vi "PAN_ModCaller.vi"(0 "CmdStringIn":string, 1 "modpath":path, 11 "error in (no error)":errorcluster) -> (4 "ImmedReplyString":string, 6 "new mod":bool, 15 "error out":errorcluster)   [LabVIEW 2016]
panel:
  in  "AVAPP Cmd Proc":refnum<vi>
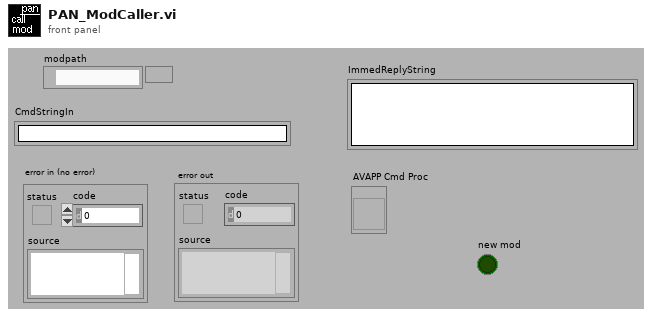
[diagram p1: front panel]
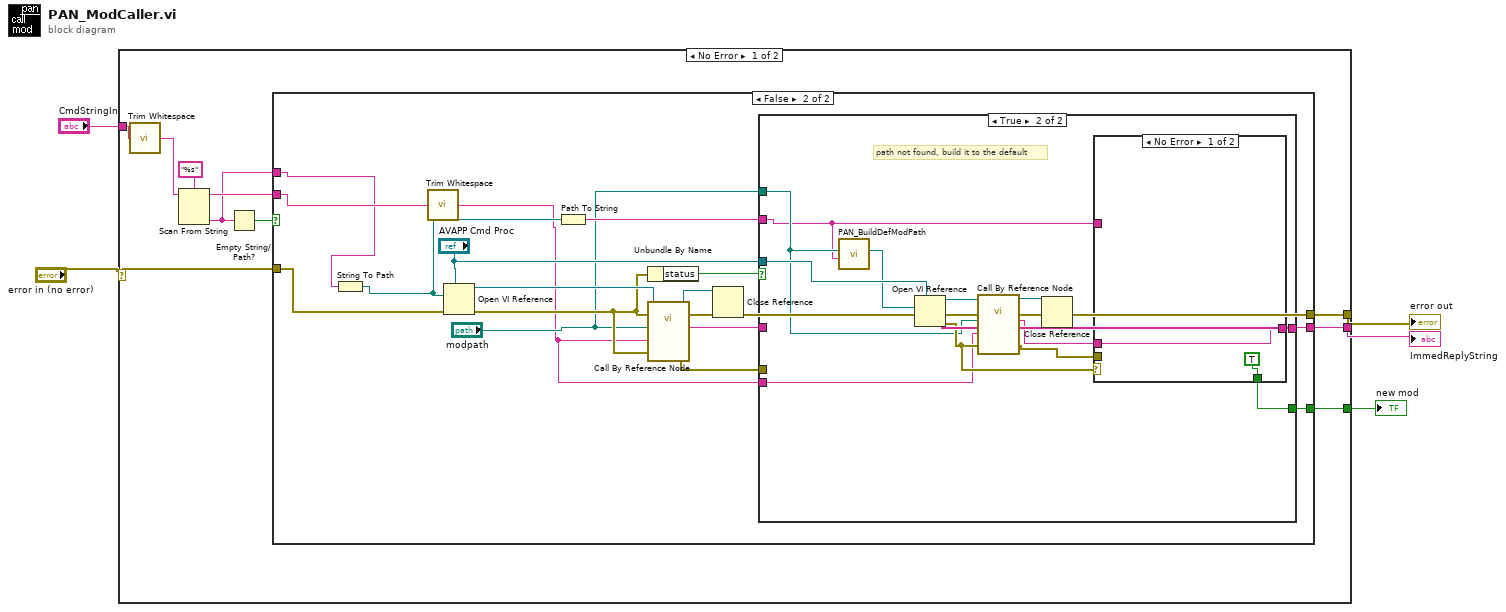
[diagram p0: block diagram]
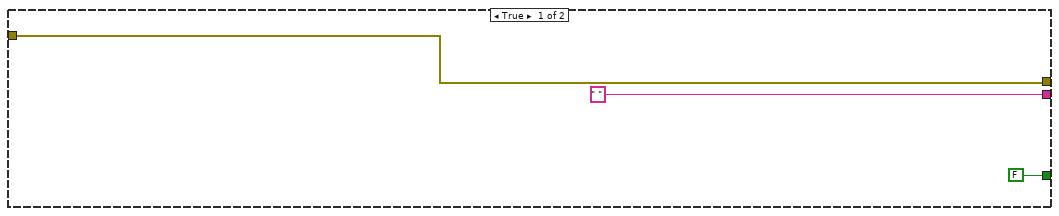
[diagram p2: hidden frame]
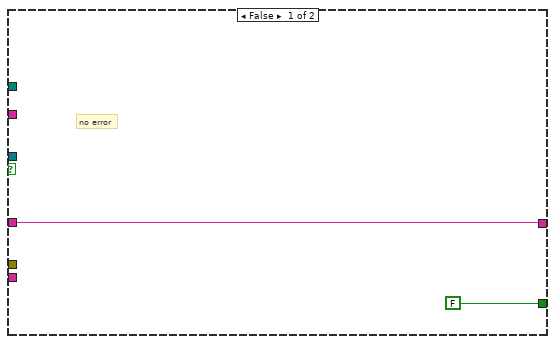
[diagram p3: hidden frame]
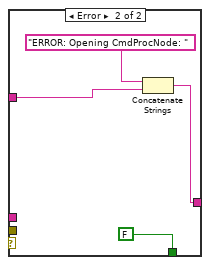
[diagram p4: hidden frame]
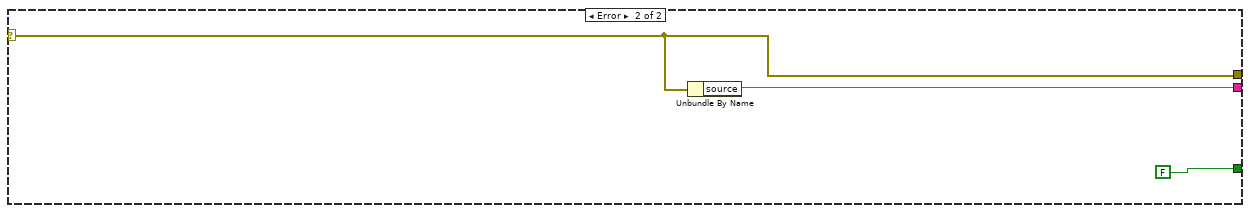
[diagram p5: hidden frame]
diagram:
  n1 = case shown="No Error" "error in (no error)" {
    selector: "error in (no error)" -> [w8 w59]
    tunnel: [w15 w58] -> w5
    tunnel: [w14 w59] -> w4
    tunnel: "CmdStringIn" -> [w13 _]
    tunnel: [w6 FALSE ("new mod")] -> w1
    frame No Error {
      n2 = call <vilib>:"Trim Whitespace.vi"("string"=w13) -> ("trimmed string"=w12:string)  [unwired: 1 in]
      n3 = Scan From String(format string="%s", input string=w12) -> (remaining string=w9:string, output 1=w7:string)  [unwired: 2 in, 3 out]
      n4 = Empty String/Path?(string/path=w7) -> (empty?=w10:bool)
      n5 = case shown="False" w10 {
        tunnel: [" " w30] -> w15
        tunnel: [w18 w32] -> w14
        tunnel: w8 -> [w18 w35]
        tunnel: w9 -> [_ w26]
        tunnel: w7 -> [_ w22]
        tunnel: [FALSE ("new mod") w19] -> w6
        frame True {
        }
        frame False {
          n6 = String To Path(string=w22) -> (path=w25:path)
          n7 = call <vilib>:"Trim Whitespace.vi"("string"=w26) -> ("trimmed string"=w20:string)  [unwired: 1 in]
          n8 = Open VI Reference(type specifier VI Refnum (for type only)="AVAPP Cmd Proc", vi path=w25, error in (no error)=w35) -> (vi reference=w36:refnum<vi>, error out=w27:errorcluster)  [unwired: 3 out]
          n9 = Path To String(path=w25) -> (string=w24:string)
          n10 = Unbundle By Name(w27) -> ("status"=w31:bool)
          n11 = call-by-ref "Call By Reference Node"(reference=w36, error in=w27, "modpath"="modpath", "Cmd"=w20, "error in"=w27) -> (reference out=w33:refnum<vi>, error out=w34:errorcluster, "ImmedReplyString"=w29:string, 15:"error out"=w28:errorcluster)  [unwired: 11 in]
          n12 = Close Reference(reference=w33, error in (no error)=w34) -> (error out=w32:errorcluster)
          n13 = case shown="True" w31 {
            tunnel: w24 -> [_ w40]
            tunnel: [w38 w50] -> w30
            tunnel: w29 -> [w38 _]
            tunnel: w28 -> [_ _]
            tunnel: "AVAPP Cmd Proc" -> [_ w48]
            tunnel: "modpath" -> [_ w41]
            tunnel: w20 -> [_ w43]
            tunnel: [FALSE ("new mod") w42] -> w19
            frame False {
              # "no error"
            }
            frame True {
              # "path not found, build it to the default"
              n14 = call "PAN_BuildDefModPath.vi"("mod name"=w40, "modpath"=w41) -> ("modapipath"=w39:path)  [unwired: 9 out]
              n15 = Open VI Reference(type specifier VI Refnum (for type only)=w48, vi path=w39) -> (vi reference=w49:refnum<vi>, error out=w46:errorcluster)  [unwired: 1 in, 3 out]
              n16 = call-by-ref "Call By Reference Node"(reference=w49, "modpath"=w41, "Cmd"=w43, "error in"=w46) -> (reference out=w47:refnum<vi>, "ImmedReplyString"=w45:string, "error out"=w44:errorcluster)  [unwired: 12 in, 1 out]
              n17 = Close Reference(reference=w47) -> ()  [unwired: 1 in, 1 out]
              n18 = case shown="No Error" w46 {
                tunnel: [w52 w55] -> w50
                tunnel: w40 -> [_ w54]
                tunnel: w45 -> [w52 _]
                tunnel: w44 -> [_ _]
                tunnel: [TRUE ("new mod") FALSE ("new mod")] -> w42
                frame No Error {
                }
                frame Error {
                  n19 = Concatenate Strings("ERROR: Opening CmdProcNode: " ("t"), w54) -> (w55:string)
                }
              }
            }
          }
        }
      }
    }
    frame Error {
      n20 = Unbundle By Name(w59) -> ("source"=w58:string)
    }
  }
  "ImmedReplyString" <- w5
  "error out" <- w4
  "new mod" <- w1
